vi "VersionCompare.vi"(9 "UpdatesFile":path) -> (1 "UpdateAvailable":bool, 2 "NewVersion":string)   [LabVIEW 2015]
uses:
  <vilib>/regexp/Match Regular Expression.xnode
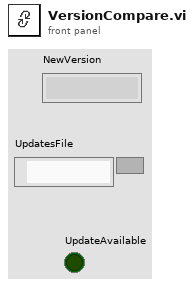
[diagram p1: front panel]
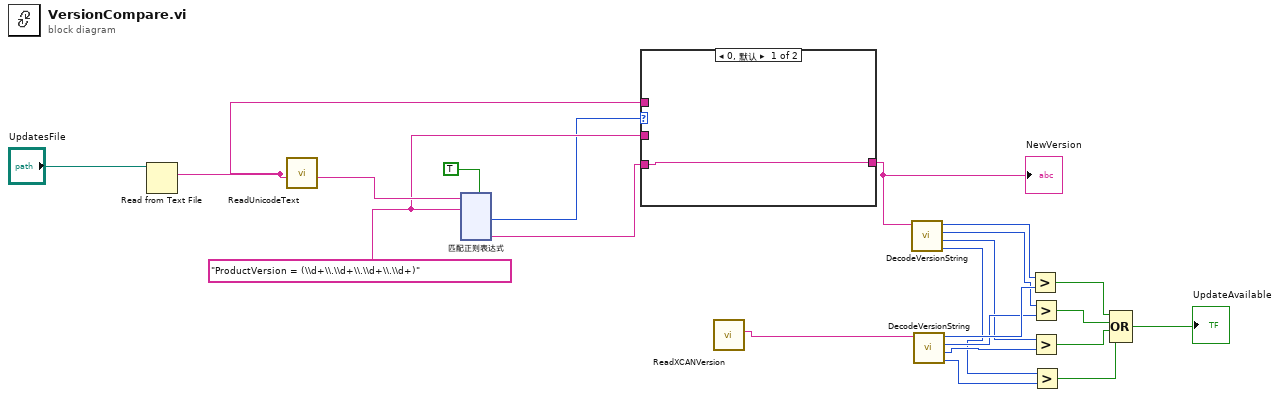
[diagram p0: block diagram]
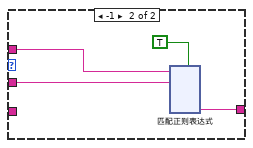
[diagram p2: hidden frame]
diagram:
  w4 = "ProductVersion = (\\d+\\.\\d+\\.\\d+\\.\\d+)" ("正则表达式")
  n1 = Read from Text File(file (use dialog)="UpdatesFile") -> (text=w5:string)  [unwired: 3 in, 3 out]
  n2 = call "ReadUnicodeText.vi"("txtIn"=w5) -> ("result string"=w20:string)  [unwired: 9 in]
  n3 = xnode "匹配正则表达式"("输入字符串"=w20, "正则表达式"=w4, "多行？(F)"=TRUE) -> ("匹配后偏移量"=w3:i32, "子匹配 1"=w1:string)  [unwired: 3 in, 4 out]
  n4 = case shown="0, 默认" w3 {
    tunnel: w5 -> [_ w26]
    tunnel: w4 -> [_ w25]
    tunnel: [w23 w24] -> w2
    tunnel: w1 -> [w23 _]
    frame 0, Default {
    }
    frame -1 {
      n5 = xnode "匹配正则表达式"("输入字符串"=w26, "正则表达式"=w25, "多行？(F)"=TRUE) -> ("子匹配 1"=w24:string)  [unwired: 3 in, 5 out]
    }
  }
  "NewVersion" <- w2
  n6 = call "ReadXCANVersion.vi"() -> ("Version"=w21:string)  [unwired: 9 in, 1 out]
  n7 = call "DecodeVersionString.vi"("VersionStr"=w2) -> ("build"=w13:i32, "correction"=w15:i32, "secondary"=w17:i32, "Main"=w19:i32)  [unwired: 5 in]
  n8 = call "DecodeVersionString.vi"("VersionStr"=w21) -> ("build"=w12:i32, "correction"=w14:i32, "secondary"=w16:i32, "Main"=w18:i32)  [unwired: 5 in]
  n9 = Greater?(x=w19, y=w18) -> (0:w11:bool)
  n10 = Greater?(x=w17, y=w16) -> (0:w9:bool)
  n11 = Greater?(x=w15, y=w14) -> (0:w10:bool)
  n12 = Greater?(x=w13, y=w12) -> (0:w8:bool)
  n13 = Compound Arithmetic op=OR ("复合运算")(w11, w9, w10, w8) -> (→"UpdateAvailable":bool)
